vi "Horizontal Bar.vi"() -> (3 "Horizontal Bar":string)   [LabVIEW 2023, in "Confluence Formatting.lvlib"]
uses:
  Confluence Formatting.lvlib
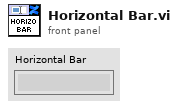
[diagram p1: front panel]
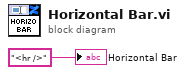
[diagram p0: block diagram]
diagram:
  "Horizontal Bar" <- "<hr />" ("Horizontal Bar")
